vi "ExWrite8BitTiff.vi"() -> ()   [LabVIEW 2010]
panel:
  in  "File Name":path
  out "error out":errorcluster
  in  "error in (no error)":errorcluster
  in  "X Size":u32=1 min=1 step=1
  in  "Y Size":u32=1 min=1 step=1
  # "NOTICE\n\nTHIS VI REQUIRES THAT THE TOOLKIT\nBE UNLOADED BY RUNNING THE\n VI EXCLOSEGLOBALCAM.VI\n BEFORE LEAVING LABVIEW."
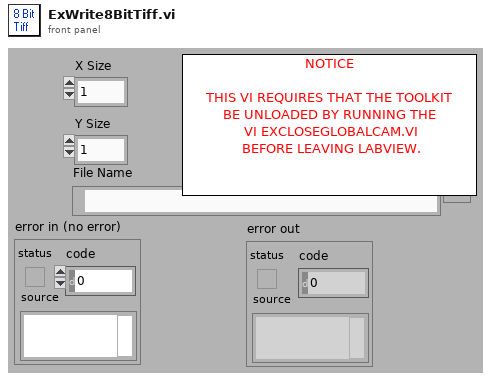
[diagram p1: front panel]
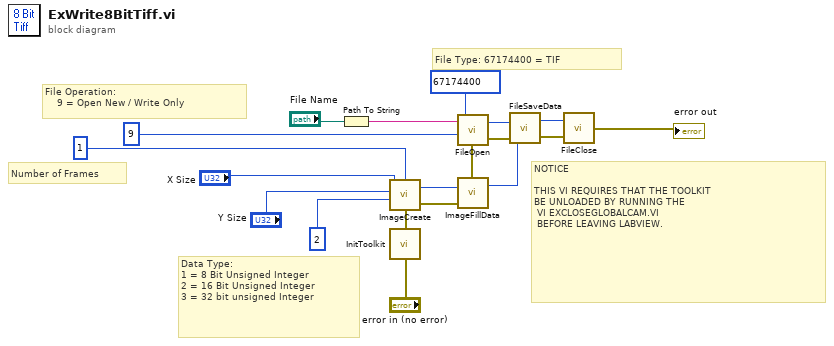
[diagram p0: block diagram]
diagram:
  # "NOTICE\n\nTHIS VI REQUIRES THAT THE TOOLKIT\nBE UNLOADED BY RUNNING THE\n VI EXCLOSEGLOBALCAM.VI\n BEFORE LEAVING LABVIEW."
  # "Data Type:\n1 = 8 Bit Unsigned Integer\n2 = 16 Bit Unsigned Integer\n3 = 32 bit unsigned Integer"
  # "File Type: 67174400 = TIF"
  # "Number of Frames"
  # "File Operation:\n    9 = Open New / Write Only"
  n1 = Path To String(path="File Name") -> (string=w2:string)
  n2 = call <userlib>:"InitToolkit.vi"("error in"="error in (no error)") -> ("error out"=w10:errorcluster)
  n3 = call <userlib>:"ImageCreate.vi"("X dimension"="X Size", "Y dimension"="Y Size", "Data Type"=u16 2, "error in"=w10, "Number Of Frames"=1) -> ("Image Handle"=w18:u32, "error out"=w19:errorcluster)
  n4 = call <userlib>:"ImageFillData.vi"("error in"=w19, "Image Handle"=w18) -> ("error out"=w13:errorcluster, "Image Handle"=w16:u32)  [unwired: 1 in]
  n5 = call <userlib>:"FileOpen.vi"("error in"=w13, "File Operations"=9, "FileName"=w2, "File Type"=67174400 ("Numeric")) -> ("error out"=w12:errorcluster, "File Handle"=w11:u32)
  n6 = call <userlib>:"FileSaveData.vi"("error in"=w12, "Image Handle"=w16, "File Handle"=w11) -> ("error out"=w17:errorcluster, "File Handle"=w15:u32)
  n7 = call <userlib>:"FileClose.vi"("error in"=w17, "File Handle"=w15) -> ("error out"=→"error out":errorcluster)
